vi "DMM Config.vi"(8 "error in (no error)":errorcluster, 9 "SMU DMM Measurement":T2, 10 "SMU Resolution in Digits":T1 items=["3 1/2"=3.5, "4 1/2"=4.5, "5 1/2"=5.5, "6 1/2"=6.5, "7 1/2"=7.5], 11 "IVI Refnum in":refnum<k15>) -> (0 "error out":errorcluster, 2 "Measurement":dbl, 3 "IVI Refnum out":refnum<k15>)   [LabVIEW 2021, in "DMM T16.lvlib"]
uses:
  DMM T16.lvlib
  <instrlib>/niDMM/nidmm.llb/niDMM Function.ctl
  <instrlib>/niDMM/nidmm.llb/niDMM Resolution in Digits.ctl
  <instrlib>/niDMM/nidmm.llb/niDMM Configure Measurement Digits.vi
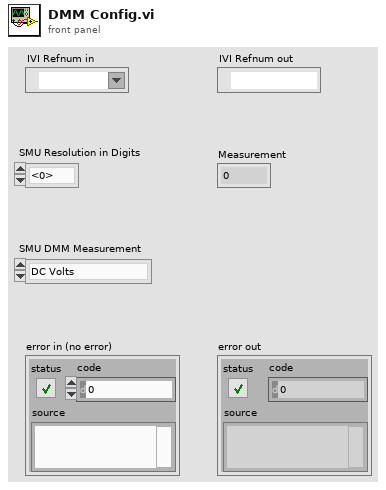
[diagram p1: front panel]
types:
  T1 = typedef "niDMM Resolution in Digits.ctl" = dbl
  T2 = typedef "niDMM Function.ctl" = enum16{"DC Volts", "AC Volts", "DC Current", "AC Current", "2-wire Resistance", "4-wire Resistance", "Diode", "Frequency", "Period", "AC Volts DC Coupled", "Capacitance", "Inductance", "Temperature"}
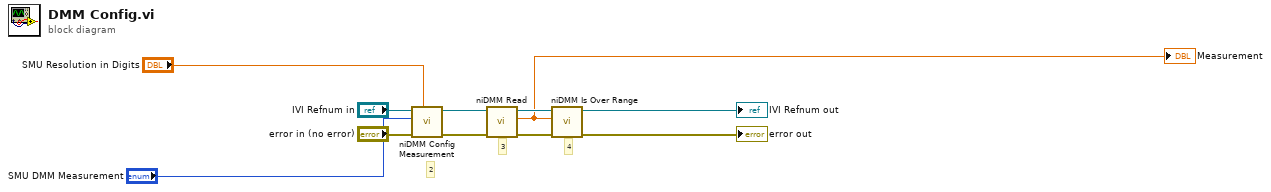
[diagram p0: block diagram]
diagram:
  # "2"
  # "4"
  # "3"
  n1 = call-poly <instrlib>:"niDMM Config Measurement.vi"("Resolution in Digits"="SMU Resolution in Digits", "error in (no error)"="error in (no error)", "Function"="SMU DMM Measurement", "instrument handle"="IVI Refnum in") -> ("error out"=w10:errorcluster, "instrument handle out"=w9:refnum<k15>)  [unwired: 6 in]
  n2 = call <instrlib>:"niDMM Read.vi"("error in (no error)"=w10, "instrument handle"=w9) -> ("error out"=w7:errorcluster, "Measurement"=w6:dbl, "instrument handle out"=w8:refnum<k15>)  [unwired: 7 in]
  "Measurement" <- w6
  n3 = call <instrlib>:"niDMM Is Over Range.vi"("error in (no error)"=w7, "Measurement"=w6, "instrument handle"=w8) -> ("error out"=→"error out":errorcluster, "instrument handle out"=→"IVI Refnum out":refnum<k15>)  [unwired: 6 in, 1 out]
